vi "Offset Table Headers.vi"(6 "Rigid Connection":bool, 7 "Coordinate Space":bool caption="Coord", 9 "Number of\nLBCBs":T1, 10 "Size":T2, 11 "Offset Type":T3=enum."External Sensors") -> (1 "Column Headers":string[](array[string]), 3 "Row Headers":string[](array[string])=["Offset", "Current"])   [LabVIEW 2009]
uses:
  Offset Types.ctl
  Data Access Objects/Metadata/LBCB Size.ctl
  Data Access Objects/Application/Number Of LBCBs.ctl
  Global Data/Name Actions.ctl
panel:
  in  "Row Header\nRoot":string[](array[string])=["Offset", "Current"]
  in  "Cartesian\nForce":string[](array[string])=["Fx", "Fy", "Fz", "Mx", "My", "Mz"]
  in  "Cartesian\nDisp":string[](array[string])=["Dx", "Dy", "Dz", "Rx", "Ry", "Rz"]
  in  "Actuators":string[](array[string])=["X1", "X2", "Y1", "Z1", "Z2", "Z3"]
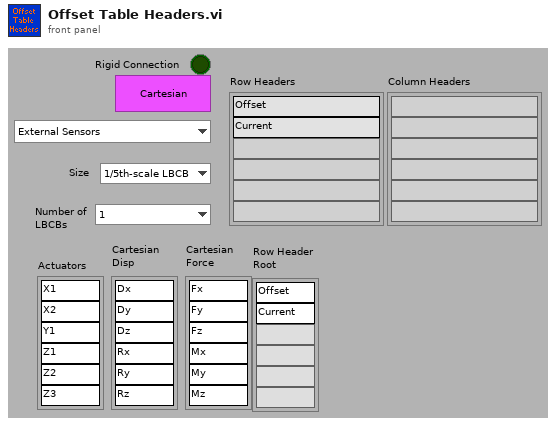
[diagram p1: front panel]
types:
  T1 = typedef "Number Of LBCBs.ctl" = enum16{"1", "2"}
  T2 = typedef "LBCB Size.ctl" = enum16{"1/5th-scale LBCB", "Full-scale LBCB", "Portable LBCB"}
  T3 = typedef "Offset Types.ctl" = enum16{"Displacements", "Forces", "External Sensors"}
  T4 = typedef "Name Actions.ctl" = enum16{"Init", "Get Names", "Get Index"}
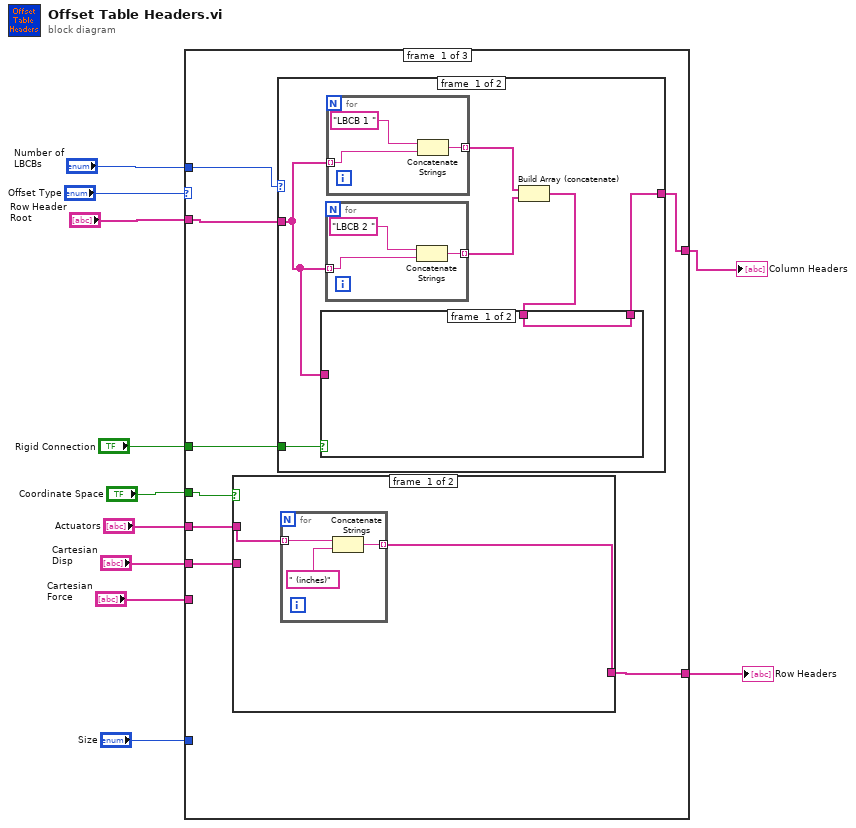
[diagram p0: block diagram]
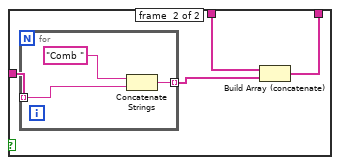
[diagram p2: hidden frame]
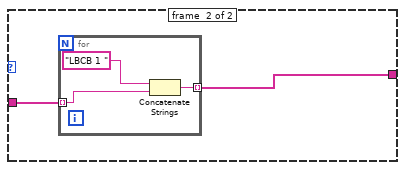
[diagram p3: hidden frame]
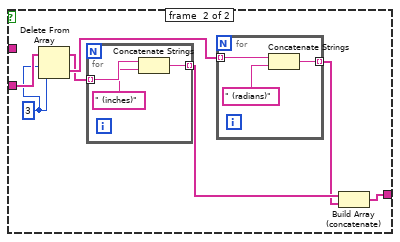
[diagram p4: hidden frame]
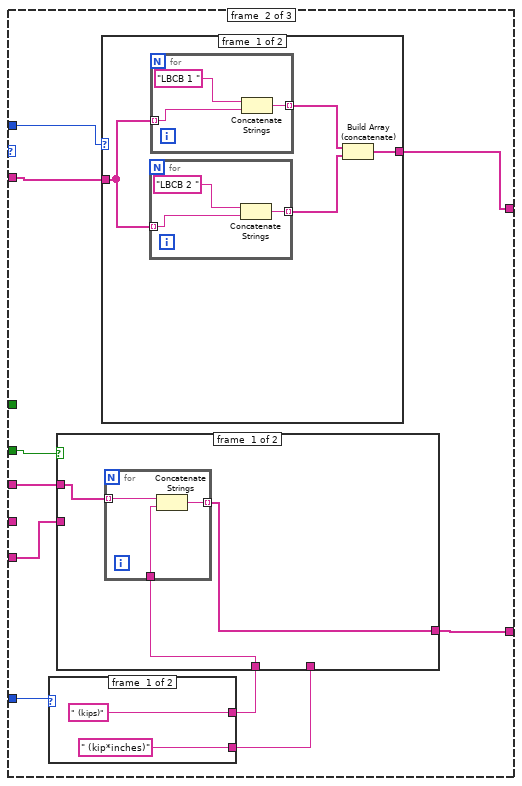
[diagram p5: hidden frame]
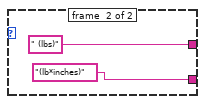
[diagram p6: hidden frame]
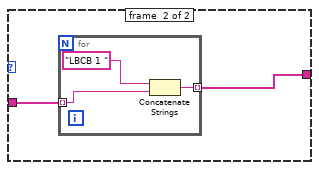
[diagram p7: hidden frame]
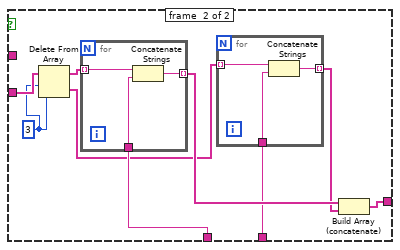
[diagram p8: hidden frame]
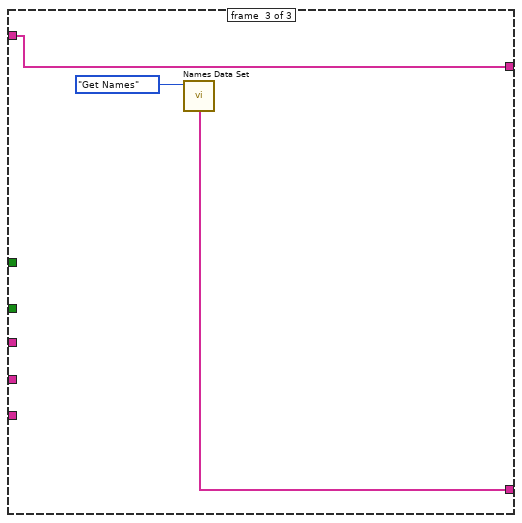
[diagram p9: hidden frame]
diagram:
  n1 = case shown="\"Displacements\"" "Offset Type" {
    tunnel: [w17 w70 w114] -> w1
    tunnel: [w14 w67 w113] -> w2
    tunnel: "Coordinate Space" -> [w19 w72 _]
    tunnel: "Actuators" -> [w18 w71 _]
    tunnel: "Row Header\nRoot" -> [w16 w69 w113]
    tunnel: "Number of\nLBCBs" -> [w15 w68 _]
    tunnel: "Cartesian\nDisp" -> [w13 _ _]
    tunnel: "Cartesian\nForce" -> [_ w66 _]
    tunnel: "Size" -> [_ w64 _]
    tunnel: "Rigid Connection" -> [w12 _ _]
    frame #0 {
      n2 = case shown="False" w19 {
        tunnel: w18 -> [w46 _]
        tunnel: [w45 w54] -> w17
        tunnel: w13 -> [_ w53]
        frame #0 {
          n3 = for {
            tunnel: w46 -> [w49] mode=indexing
            tunnel: [w47] -> w45 mode=indexing
            n4 = Concatenate Strings(w49, " (inches)") -> (w47:string)
          }
        }
        frame #1 {
          w52 = 3 ("index")
          n5 = Delete From Array(array=w53, length=w52, index=w52) -> (deleted portion=w51:string[], array with subset deleted=w50:string[])
          n6 = for {
            tunnel: w50 -> [w62] mode=indexing
            tunnel: [w60] -> w56 mode=indexing
            n7 = Concatenate Strings(w62, " (inches)") -> (w60:string)
          }
          n8 = for {
            tunnel: w51 -> [w59] mode=indexing
            tunnel: [w57] -> w55 mode=indexing
            n9 = Concatenate Strings(w59, " (radians)") -> (w57:string)
          }
          n10 = Build Array (concatenate)(w56, w55) -> (w54:string[])
        }
      }
      n11 = case shown="\"2\"" w15 {
        tunnel: w16 -> [w23 w41]
        tunnel: [w20 w40] -> w14
        tunnel: w12 -> [w22 _]
        frame #0 {
          n12 = for {
            tunnel: w23 -> [w39] mode=indexing
            tunnel: [w37] -> w24 mode=indexing
            n13 = Concatenate Strings("LBCB 2 " ("string"), w39) -> (w37:string)
          }
          n14 = for {
            tunnel: w23 -> [w36] mode=indexing
            tunnel: [w34] -> w25 mode=indexing
            n15 = Concatenate Strings("LBCB 1 " ("string"), w36) -> (w34:string)
          }
          n16 = Build Array (concatenate)(w25, w24) -> (w21:string[])
          n17 = case shown="True" w22 {
            tunnel: w23 -> [_ w30]
            tunnel: w21 -> [w26 w29]
            tunnel: [w26 w27] -> w20
            frame #0 {
            }
            frame #1 {
              n18 = for {
                tunnel: w30 -> [w33] mode=indexing
                tunnel: [w31] -> w28 mode=indexing
                n19 = Concatenate Strings("Comb " ("string"), w33) -> (w31:string)
              }
              n20 = Build Array (concatenate)(w29, w28) -> (w27:string[])
            }
          }
        }
        frame #1 {
          n21 = for {
            tunnel: w41 -> [w44] mode=indexing
            tunnel: [w42] -> w40 mode=indexing
            n22 = Concatenate Strings("LBCB 1 " ("string"), w44) -> (w42:string)
          }
        }
      }
    }
    frame #1 {
      n23 = case shown="\"1/5th-scale LBCB\", Default" w64 {
        tunnel: [" (kips)" " (lbs)"] -> w65
        tunnel: [" (kip*inches)" "(lb*inches)"] -> w63
        frame #0 {
        }
        frame #1 {
        }
      }
      n24 = case shown="False" w72 {
        tunnel: w71 -> [w94 _]
        tunnel: [w93 w104] -> w70
        tunnel: w66 -> [_ w101]
        tunnel: w65 -> [w92 w103]
        tunnel: w63 -> [_ w102]
        frame #0 {
          n25 = for {
            tunnel: w94 -> [w97] mode=indexing
            tunnel: [w96] -> w93 mode=indexing
            tunnel: w92 -> [w95]
            n26 = Concatenate Strings(w97, w95) -> (w96:string)
          }
        }
        frame #1 {
          w98 = 3 ("index")
          n27 = Delete From Array(array=w101, length=w98, index=w98) -> (deleted portion=w99:string[], array with subset deleted=w100:string[])
          n28 = for {
            tunnel: w100 -> [w112] mode=indexing
            tunnel: [w111] -> w106 mode=indexing
            tunnel: w103 -> [w110]
            n29 = Concatenate Strings(w112, w110) -> (w111:string)
          }
          n30 = for {
            tunnel: w99 -> [w109] mode=indexing
            tunnel: [w108] -> w105 mode=indexing
            tunnel: w102 -> [w107]
            n31 = Concatenate Strings(w109, w107) -> (w108:string)
          }
          n32 = Build Array (concatenate)(w106, w105) -> (w104:string[])
        }
      }
      n33 = case shown="\"1\"" w68 {
        tunnel: w69 -> [w80 w88]
        tunnel: [w77 w87] -> w67
        frame #0 {
          n34 = for {
            tunnel: w80 -> [w86] mode=indexing
            tunnel: [w84] -> w78 mode=indexing
            n35 = Concatenate Strings("LBCB 2 " ("string"), w86) -> (w84:string)
          }
          n36 = for {
            tunnel: w80 -> [w83] mode=indexing
            tunnel: [w81] -> w79 mode=indexing
            n37 = Concatenate Strings("LBCB 1 " ("string"), w83) -> (w81:string)
          }
          n38 = Build Array (concatenate)(w79, w78) -> (w77:string[])
        }
        frame #1 {
          n39 = for {
            tunnel: w88 -> [w91] mode=indexing
            tunnel: [w89] -> w87 mode=indexing
            n40 = Concatenate Strings("LBCB 1 " ("string"), w91) -> (w89:string)
          }
        }
      }
    }
    frame #2 {
      n41 = call "Names Data Set.vi"("Name Actions"=Name_Actions."Get Names") -> ("External Sensor Names"=w114:string[])  [unwired: 1 in, 13 out]
    }
  }
  "Row Headers" <- w1
  "Column Headers" <- w2
